vi "FormatIntoString2.vi"() -> ()   [LabVIEW 2019]
panel:
  out "Output":string
  in  "Thermometer":dbl(slide) scale=0.0..100.0
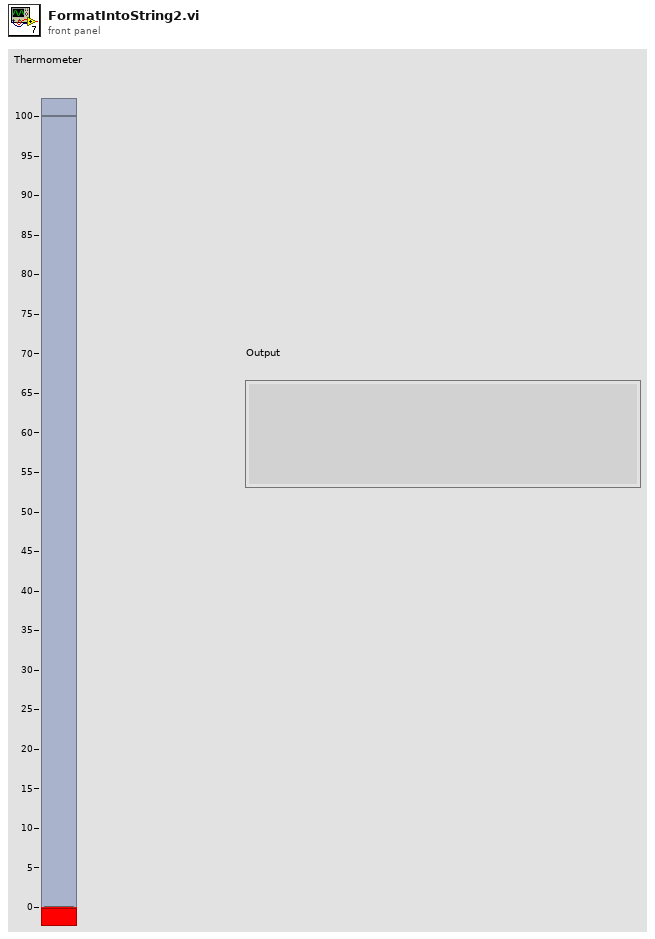
[diagram p1: front panel]
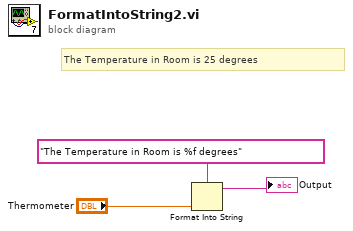
[diagram p0: block diagram]
diagram:
  # "The Temperature in Room is 25 degrees"
  n1 = Format Into String(format string="The Temperature in Room is %f degrees", "Thermometer") -> (resulting string=→"Output":string)  [unwired: 2 in, 1 out]
